vi "Metadata Test.vi"() -> ()   [LabVIEW 2019, in "metadata.lvclass"]
uses:
  metadata.lvclass
  File info parameters.ctl
  System control parameters.ctl
  Sample info parameters.ctl
  Cantilever info parameters.ctl
  XYZ piezos parameters.ctl
  Mapping parameters.ctl
  Fcurve segment.ctl
  Segment type--combobox.ctl
  fast fpga segment parameters.ctl
  Chirp added parameters.ctl
panel:
  out "String":string
  out "Metadata":T1
  out "Post Metadat Fcurve":string
  in  "Chirp input":T2[](array[typedef])
  in  "Fast FPGA intput":T3[](array[typedef])
  in  "Force curve segments":T4[](array[typedef])
  in  "Mapping":T6
  in  "XYZ piezos":T7
  in  "Cantilever info":T8
  in  "Sample info":T9
  in  "System Control":T10
  in  "file info":T11
  out "Pre Metadat Fcurve":string
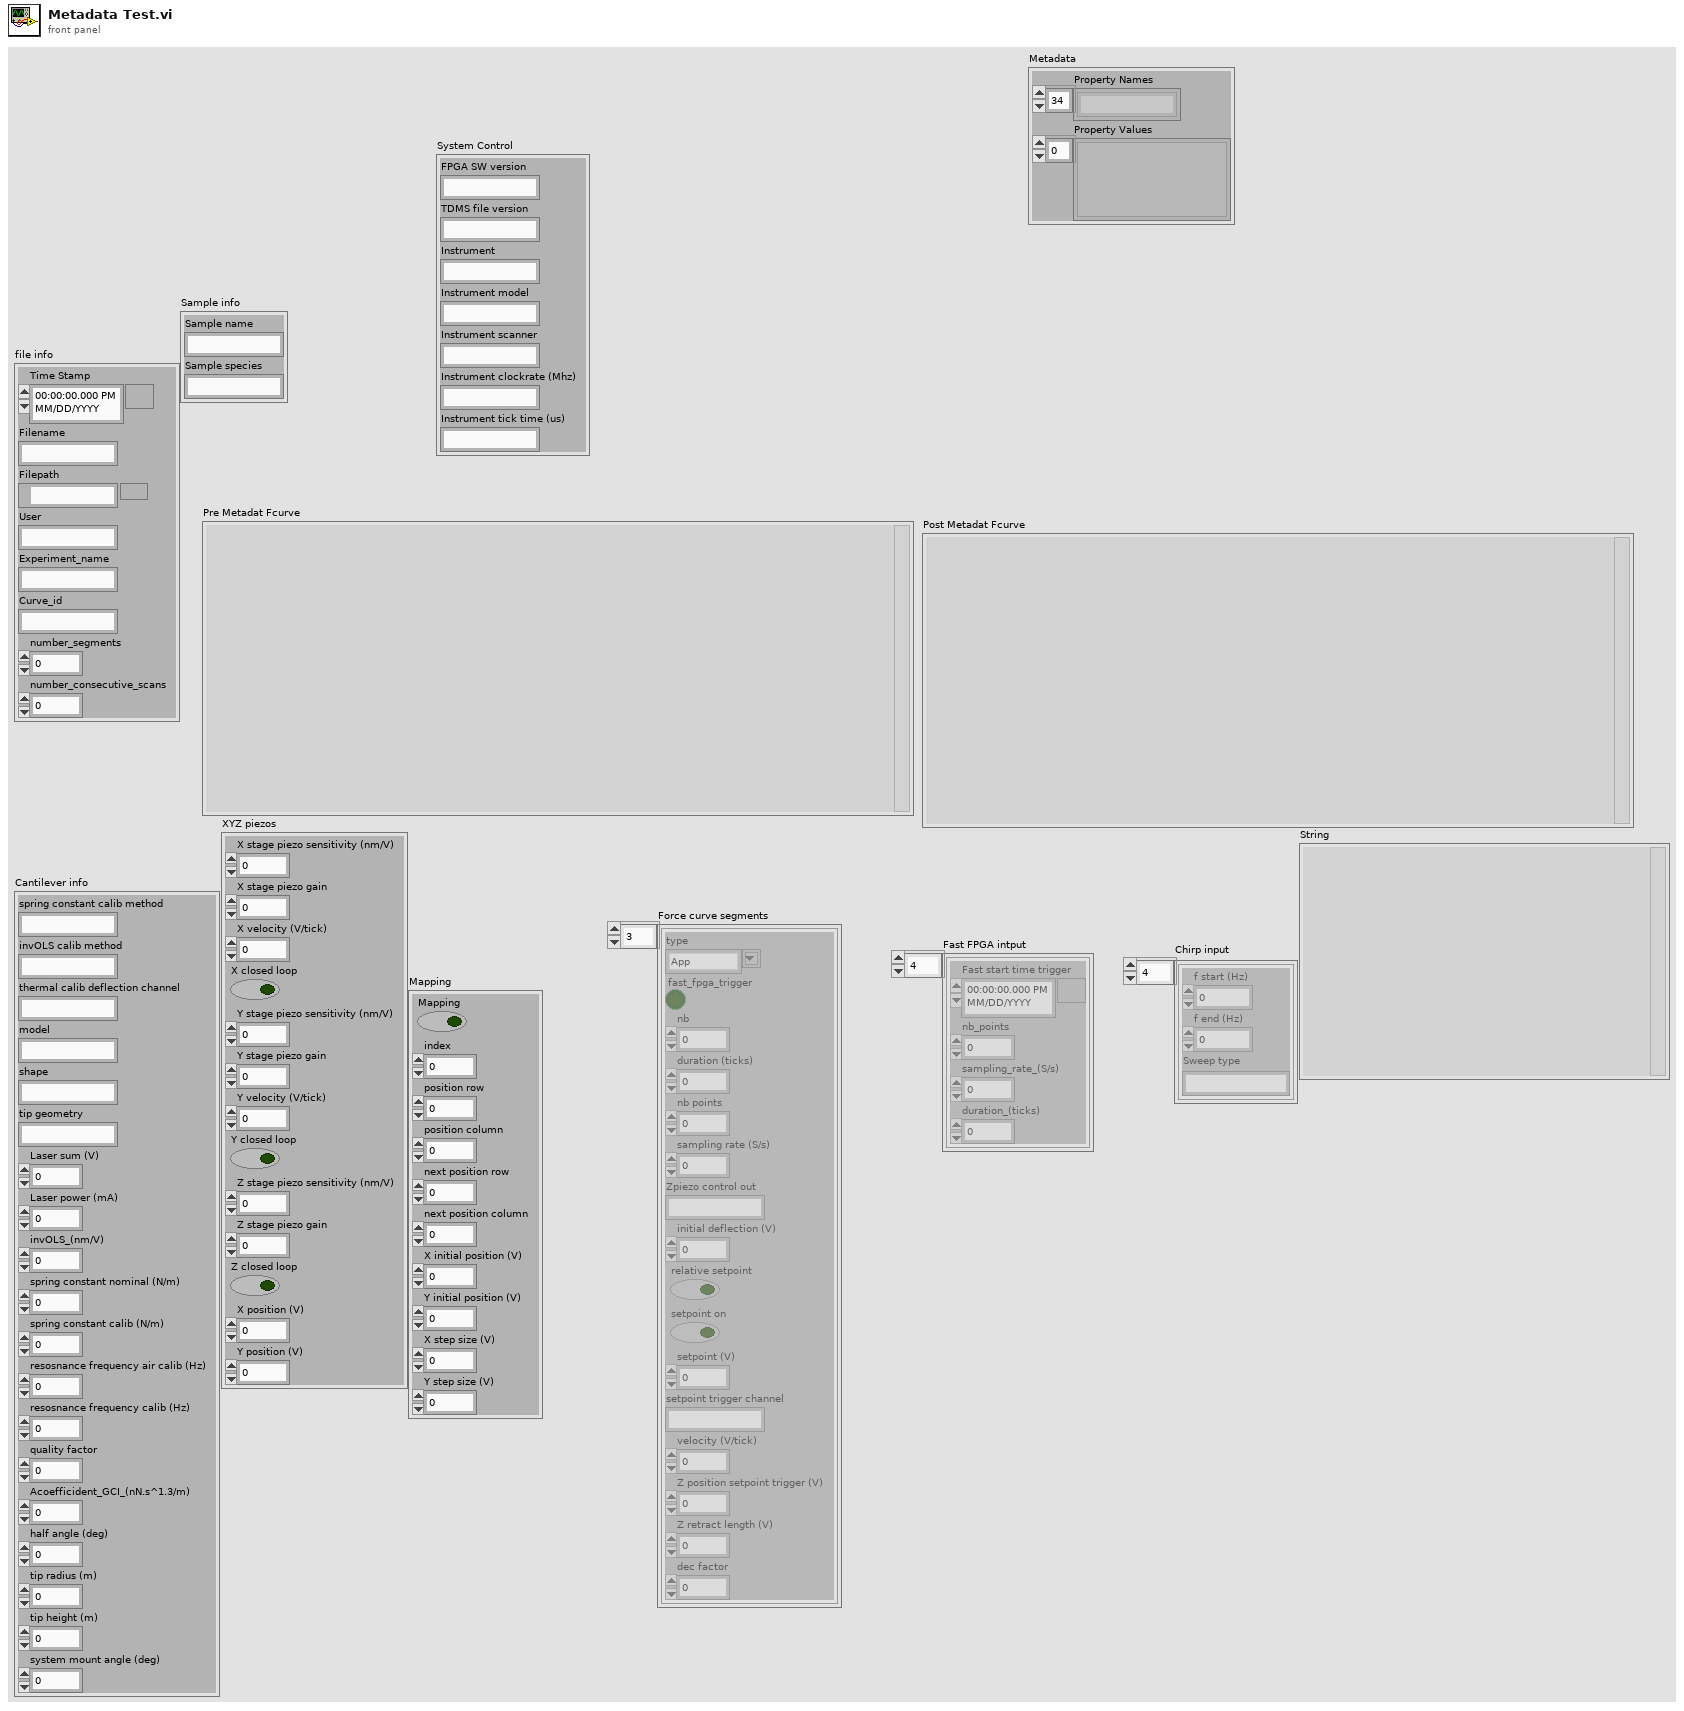
[diagram p1: front panel]
types:
  T1 = cluster{"Property Names":string[], "Property Values":variant[]}
  T2 = typedef "metadata.lvclass/Chirp added parameters.ctl" = cluster{"f start (Hz)":dbl, "f end (Hz)":dbl, "Sweep type":string}
  T3 = typedef "metadata.lvclass/fast fpga segment parameters.ctl" = cluster{"Fast start time trigger":timestamp, "nb_points":u32, "sampling_rate_(S/s)":u32, "duration_(ticks)":u32}
  T4 = typedef "metadata.lvclass/Fcurve segment.ctl" = cluster{"type":T5, "fast_fpga_trigger":bool, "nb":u8, "duration (ticks)":i64, "nb points":i32, "sampling rate (S/s)":u32, "Zpiezo control out":string, "initial deflection (V)":dbl, "relative setpoint":bool, "setpoint on":bool, "setpoint (V)":dbl, "setpoint trigger channel":string, "velocity (V/tick)":dbl, "Z position setpoint trigger (V)":dbl, "Z retract length (V)":dbl, "dec factor":u32}
  T5 = typedef "metadata.lvclass/Segment type--combobox.ctl" = string
  T6 = typedef "metadata.lvclass/Mapping parameters.ctl" = cluster{"Mapping":bool, "index":u16, "position row":u16, "position column":u16, "next position row":i16, "next position column":i16, "X initial position (V)":dbl, "Y initial position (V)":dbl, "X step size (V)":dbl, "Y step size (V)":dbl}
  T7 = typedef "metadata.lvclass/XYZ piezos parameters.ctl" = cluster{"X stage piezo sensitivity (nm/V)":dbl, "X stage piezo gain":dbl, "X velocity (V/tick)":dbl, "X closed loop":bool, "Y stage piezo sensitivity (nm/V)":dbl, "Y stage piezo gain":dbl, "Y velocity (V/tick)":dbl, "Y closed loop":bool, "Z stage piezo sensitivity (nm/V)":dbl, "Z stage piezo gain":dbl, "Z closed loop":bool, "X position (V)":dbl, "Y position (V)":dbl}
  T8 = typedef "metadata.lvclass/Cantilever info parameters.ctl" = cluster{"spring constant calib method":string, "invOLS calib method":string, "thermal calib deflection channel":string, "model":string, "shape":string, "tip geometry":string, "Laser sum (V)":dbl, "Laser power (mA)":dbl, "invOLS_(nm/V)":dbl, "spring constant nominal (N/m)":dbl, "spring constant calib (N/m)":dbl, "resosnance frequency air calib (Hz)":dbl, "resosnance frequency calib (Hz)":dbl, "quality factor":dbl, "Acoefficident_GCI_(nN.s^1.3/m)":dbl, "half angle (deg)":dbl, "tip radius (m)":dbl, "tip height (m)":dbl, "system mount angle (deg)":dbl}
  T9 = typedef "metadata.lvclass/Sample info parameters.ctl" = cluster{"Sample name":string, "Sample species":string}
  T10 = typedef "metadata.lvclass/System control parameters.ctl" = cluster{"FPGA SW version":string, "TDMS file version":string, "Instrument":string, "Instrument model":string, "Instrument scanner":string, "Instrument clockrate (Mhz)":string, "Instrument tick time (us)":string}
  T11 = typedef "metadata.lvclass/File info parameters.ctl" = cluster{"Time Stamp":timestamp, "Filename":string, "Filepath":path, "User":string, "Experiment_name":string, "Curve_id":string, "number_segments":u8, "number_consecutive_scans":u32}
  T12 = typedef "metadata.lvclass/Metadata output --cluster.ctl" = cluster{"Property Names":string[], "Property Values":variant[]}
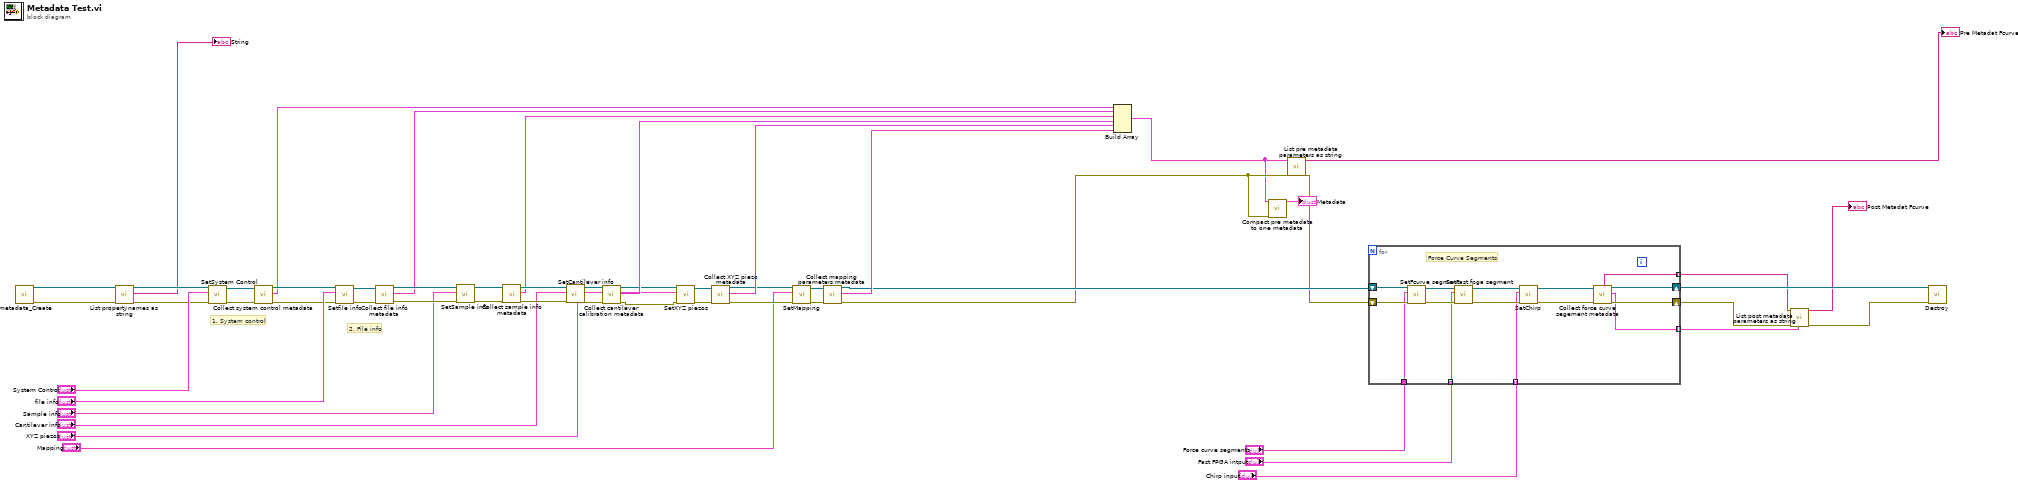
[diagram p0: block diagram]
diagram:
  # "2. File info"
  # "1. System control"
  n1 = call "metadata_Create.vi"() -> ("reference out"=w54:refnum<class "metadata.lvclass">, "error out"=w53:errorcluster)  [unwired: 18 in]
  n2 = call "List propertynames as string.vi"("reference in"=w54, "error in (no error)"=w53) -> ("reference out"=w3:refnum<class "metadata.lvclass">, "String"=→"String":string, "error out"=w2:errorcluster)  [unwired: 15 in]
  n3 = call-dynamic "SetSystem Control.vi"("error in (no error)"=w2, "System Control"="System Control", "reference in"=w3) -> ("error out"=w47:errorcluster, "reference out"=w49:refnum<class "metadata.lvclass">)  [unwired: 7 in]
  n4 = call-dynamic "Collect system control metadata.vi"("reference in"=w49, "error in (no error)"=w47) -> ("reference out"=w48:refnum<class "metadata.lvclass">, "Metadata"=w34:T12, "error out"=w46:errorcluster)  [unwired: 15 in]
  n5 = call-dynamic "Setfile info.vi"("error in (no error)"=w46, "file info"="file info", "reference in"=w48) -> ("error out"=w50:errorcluster, "reference out"=w51:refnum<class "metadata.lvclass">)  [unwired: 7 in]
  n6 = call-dynamic "Collect file info metadata.vi"("reference in"=w51, "error in (no error)"=w50) -> ("reference out"=w44:refnum<class "metadata.lvclass">, "Metadata"=w33:T12, "error out"=w42:errorcluster)  [unwired: 15 in]
  n7 = call-dynamic "SetSample info.vi"("error in (no error)"=w42, "Sample info"="Sample info", "reference in"=w44) -> ("error out"=w40:errorcluster, "reference out"=w43:refnum<class "metadata.lvclass">)  [unwired: 7 in]
  n8 = call-dynamic "Collect sample info metadata.vi"("reference in"=w43, "error in (no error)"=w40) -> ("reference out"=w39:refnum<class "metadata.lvclass">, "Metadata"=w32:T12, "error out"=w38:errorcluster)  [unwired: 15 in]
  n9 = call-dynamic "SetCantilever info.vi"("error in (no error)"=w38, "Cantilever info"="Cantilever info", "reference in"=w39) -> ("error out"=w36:errorcluster, "reference out"=w35:refnum<class "metadata.lvclass">)  [unwired: 7 in]
  n10 = call-dynamic "Collect cantilever calibration metadata.vi"("reference in"=w35, "error in (no error)"=w36) -> ("reference out"=w29:refnum<class "metadata.lvclass">, "Metadata"=w31:T12, "error out"=w27:errorcluster)  [unwired: 15 in]
  n11 = call-dynamic "SetXYZ piezos.vi"("error in (no error)"=w27, "XYZ piezos"="XYZ piezos", "reference in"=w29) -> ("error out"=w26:errorcluster, "reference out"=w28:refnum<class "metadata.lvclass">)  [unwired: 7 in]
  n12 = call-dynamic "Collect XYZ piezo metadata.vi"("reference in"=w28, "error in (no error)"=w26) -> ("reference out"=w24:refnum<class "metadata.lvclass">, "Metadata"=w30:T12, "error out"=w22:errorcluster)  [unwired: 15 in]
  n13 = call-dynamic "SetMapping.vi"("error in (no error)"=w22, "Mapping"="Mapping", "reference in"=w24) -> ("error out"=w21:errorcluster, "reference out"=w23:refnum<class "metadata.lvclass">)  [unwired: 7 in]
  n14 = call-dynamic "Collect mapping parameters metadata.vi"("reference in"=w23, "error in (no error)"=w21) -> ("reference out"=w17:refnum<class "metadata.lvclass">, "Metadata"=w20:T12, "error out"=w6:errorcluster)  [unwired: 15 in]
  n15 = Build Array(w34, w33, w32, w31, w30, w20) -> (w5:T12[])
  n16 = call "Compact pre metadata to one metadata.vi"("appended array"=w5, "error in (no error)"=w6) -> ("Metadata"=→"Metadata":T1)  [unwired: 16 in, 1 out]
  n17 = call "List pre metadata parameters as string.vi"("appended array"=w5, "error in (no error)"=w6) -> ("Pre Metadat Fcurve"=→"Pre Metadat Fcurve":string, "error out"=w15:errorcluster)  [unwired: 16 in]
  n18 = for {
    shift-right: [w67] -> w16
    shift-left: w17 -> [w69]
    shift-right: [w66] -> w10
    shift-left: w15 -> [w68]
    tunnel: [w59] -> w11 mode=indexing
    tunnel: "Force curve segments" -> [w55]
    tunnel: "Fast FPGA intput" -> [w58] mode=indexing
    tunnel: "Chirp input" -> [w57] mode=indexing
    tunnel: [w56] -> w8 mode=indexing
    # "Force Curve Segments"
    n19 = call-dynamic "SetFcurve segment.vi"("error in (no error)"=w68, "Fcurve segment"=w55, "reference in"=w69) -> ("error out"=w61:errorcluster, "reference out"=w63:refnum<class "metadata.lvclass">)  [unwired: 7 in]
    n20 = call-dynamic "SetFast fpga segment.vi"("error in (no error)"=w61, "Fast fpga segment"=w58, "reference in"=w63) -> ("error out"=w60:errorcluster, "reference out"=w62:refnum<class "metadata.lvclass">)  [unwired: 7 in]
    n21 = call-dynamic "SetChirp.vi"("error in (no error)"=w60, "Chirp"=w57, "reference in"=w62) -> ("error out"=w64:errorcluster, "reference out"=w65:refnum<class "metadata.lvclass">)  [unwired: 7 in]
    n22 = call-dynamic "Collect force curve segement metadata.vi"("reference in"=w65, "error in (no error)"=w64) -> ("Segment Header"=w56:string, "reference out"=w67:refnum<class "metadata.lvclass">, "Metadata"=w59:T12, "error out"=w66:errorcluster)  [unwired: 13 in, 1 out]
  }
  n23 = call "List post metadata parameters as string.vi"("section names"=w8, "error in (no error)"=w10, "appended array"=w11) -> ("Pre Metadat Fcurve"=→"Post Metadat Fcurve":string, "error out"=w9:errorcluster)  [unwired: 15 in]
  n24 = call-dynamic "Destroy.vi"("reference in"=w16, "error in (no error)"=w9) -> ()  [unwired: 16 in, 2 out]
